vi "closeport.vi"(8 "error in (no error)":errorcluster caption="entrée d'erreur (pas d'erreur)") -> (0 "error out":errorcluster caption="sortie d'erreur", 3 "function return":i32)   [LabVIEW 2020]
doc: "EXPORT int CALLBACK closeport();"
uses:
  TSCLIB.lvlib
  TSCLIB.dll
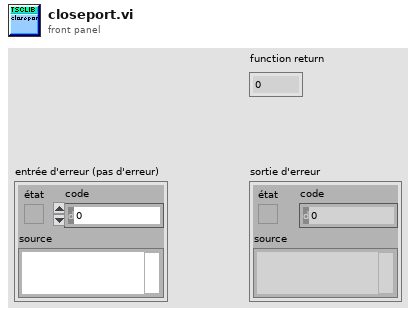
[diagram p1: front panel]
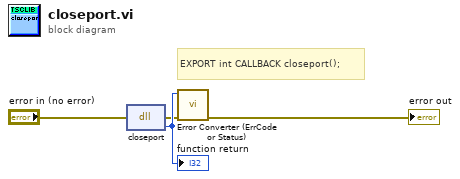
[diagram p0: block diagram]
diagram:
  # "EXPORT int CALLBACK closeport();"
  n1 = dll-call lib="C:/Users/ngarcin/OneDrive - Altyor/Standard TB/Class/Printer/Printer TSC/TSCLIB/TSCLIB.*" fn="closeport"(error in="error in (no error)") -> (error out=w2:errorcluster, "type de retour"=w4:i32)  [unwired: 2 in, 1 out]
  "function return" <- w4
  n2 = call "Error Converter (ErrCode or Status).vi"("error in (no error)"=w2, "error code"=w4) -> ("error out"=→"error out":errorcluster)  [unwired: 9 in]
